vi "InitApp.vi"(8 "ErrorArray In":errorcluster[](array[cluster]), 10 "clFrontPanelControlRefs":T1) -> (0 "ErrorArray Out":errorcluster[](array[cluster]))   [LabVIEW 2014]
uses:
  Framework.lvlib
  Apps/Typedefs/clAppData.ctl
  Bus.lvclass
  FrontPanel/TypeDefs/clEventConfig.ctl
  PmuImpairment/PmuImpairPlugins/PmuImpairPluginBase_class/TypeDefs/clImpairConfig.ctl
  PmuImpairment/PmuImpairPlugins/PmuImpairPluginBase_class/PmuImpairPluginBase.lvclass
  FrontPanel/TypeDefs/clFrontPanelControlRefs.ctl
panel:
  # "When you add a control \non the front panel, add a\nreference for it in this\ntype def.  This cluster\nwill hold all of the refer-\nences to the front panel\ncontrols in order to pass\nthese control references \nto subvis."
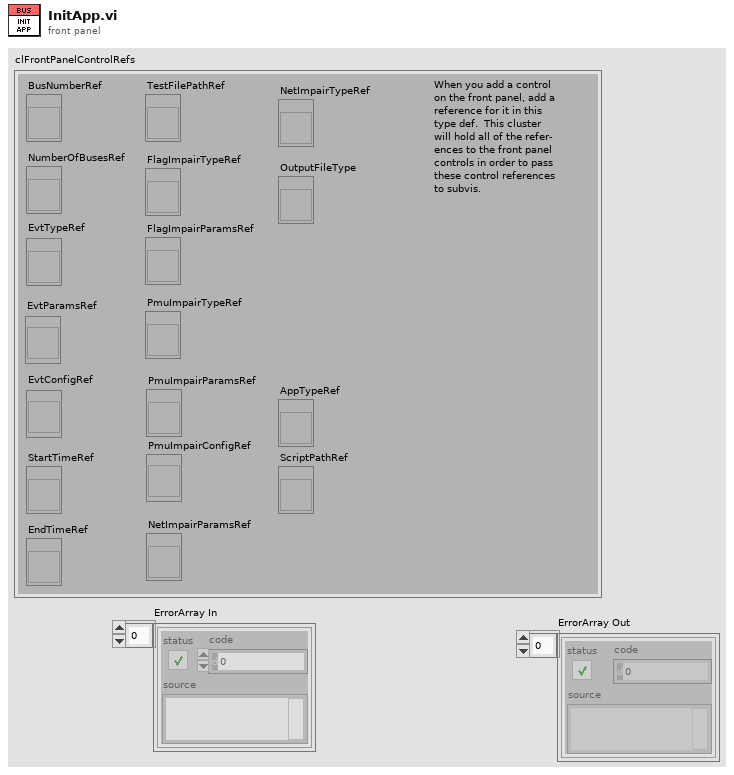
[diagram p1: front panel]
types:
  T1 = typedef "Framework.lvlib/clFrontPanelControlRefs.ctl" = cluster{"TestFilePathRef":refnum<vi>, "BusNumberRef":refnum<vi>, "NumberOfBusesRef":refnum<vi>, "EvtTypeRef":refnum<vi>, "EvtParamsRef":refnum<vi>, "EvtConfigRef":refnum<vi>, "StartTimeRef":refnum<vi>, "EndTimeRef":refnum<vi>, "PmuImpairTypeRef":refnum<vi>, "PmuImpairParamsRef":refnum<vi>, "NetImpairParamsRef":refnum<vi>, "FlagImpairTypeRef":refnum<vi>, "FlagImpairParamsRef":refnum<vi>, "NetImpairTypeRef":refnum<vi>, "OutputFileType":refnum<vi>, "PmuImpairConfigRef":refnum<vi>, "AppTypeRef":refnum<vi>, "ScriptPathRef":refnum<vi>}
  T2 = typedef "Framework.lvlib/clAppData.ctl" = cluster{"AppINIFilePath":path}
  T3 = typedef "Framework.lvlib/clFrameworkData.ctl" = cluster{"EvtINIFilePaths":path[], "BusClassInstances":refnum<class "Bus.lvclass">[], "PmuImpairINIFilePaths":path[], "FlagImpairINIFilePaths":path[], "NetImpairINIFilePaths":path[], "OutputToFileINIFilePaths":path[], "AppINIFilePaths":path[], "AppModuleID":i32, "OutputToFileID":i32}
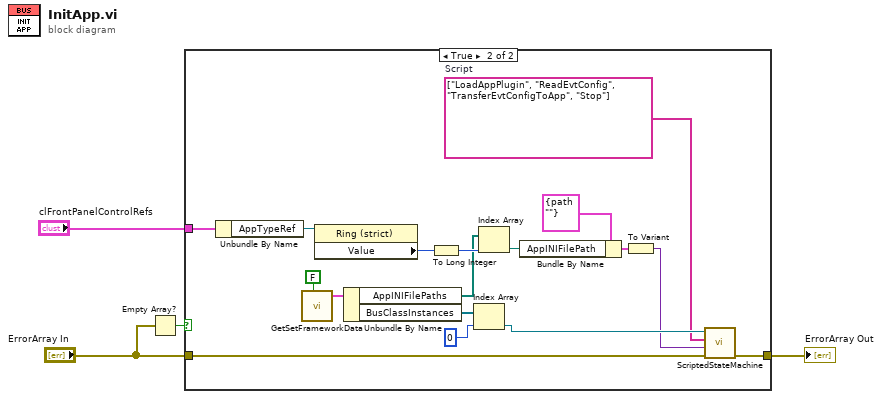
[diagram p0: block diagram]
diagram:
  n1 = Empty Array?(array="ErrorArray In") -> (empty?=w4:bool)
  n2 = case shown="True" w4 {
    tunnel: "ErrorArray In" -> [w5 w12]
    tunnel: [w5 w12] -> w3
    tunnel: "clFrontPanelControlRefs" -> [_ w21]
    frame False {
    }
    frame True {
      w6 = string[] ["LoadAppPlugin", "ReadEvtConfig", "TransferEvtConfigToApp", "Stop"]  # Script
      n3 = Unbundle By Name(w21) -> ("AppTypeRef"=w20:refnum<vi>)
      n4 = call "GetSetFrameworkData.vi"("Set (F)"=FALSE) -> ("clFrameworkData Out"=w17:T3)  [unwired: 10 in]
      n5 = property class="Ring (strict)"(reference=w20) -> ("Value"=w18:u16)  [unwired: 1 in, 2 out]
      n6 = Unbundle By Name(w17) -> ("AppINIFilePaths"=w15:path[], "BusClassInstances"=w11:refnum<class "Bus.lvclass">[])
      n7 = To Long Integer(number=w18) -> (32bit integer=w16:i32)
      n8 = Index Array(array=w11, index=0) -> (element=w9:refnum<class "Bus.lvclass">)
      n9 = Index Array(array=w15, index=w16) -> (element=w13:path)
      n10 = Bundle By Name(cluster=T2 {"AppINIFilePath"=path ""} ("clAppData"), "AppINIFilePath"=w13) -> (w8:T2)
      n11 = To Variant(anything=w8) -> (Variant=w7:variant)
      n12 = call "ScriptedStateMachine.vi"("ErrorArray In"=w12, "Data in"=w7, "Script"=w6, "Bus"=w9) -> ()  [unwired: 5 in, 3 out]
    }
  }
  "ErrorArray Out" <- w3
